vi "DXYN.vi"(11 "Variables and Memory in":T1 {"GFX" format="%02x"}) -> (3 "Variables and Memory out":T1 {"GFX" format="%02x"})   [LabVIEW 2018]
uses:
  Controls/ClusterF.ctl
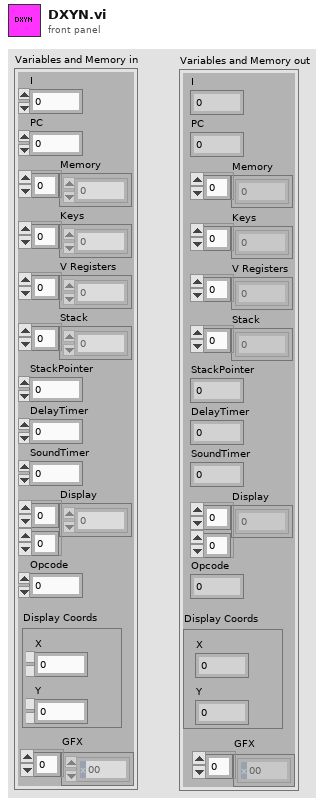
[diagram p1: front panel]
types:
  T1 = typedef "ClusterF.ctl" = cluster{"I":u16, "PC":u16, "Memory":u8[], "Keys":u8[], "V Registers":u8[], "Stack":u16[], "StackPointer":u16, "DelayTimer":u8, "SoundTimer":u8, "Display":u8[][], "Opcode":u16, "Display Coords":cluster{"X":u8, "Y":u8}, "GFX":u8[]}
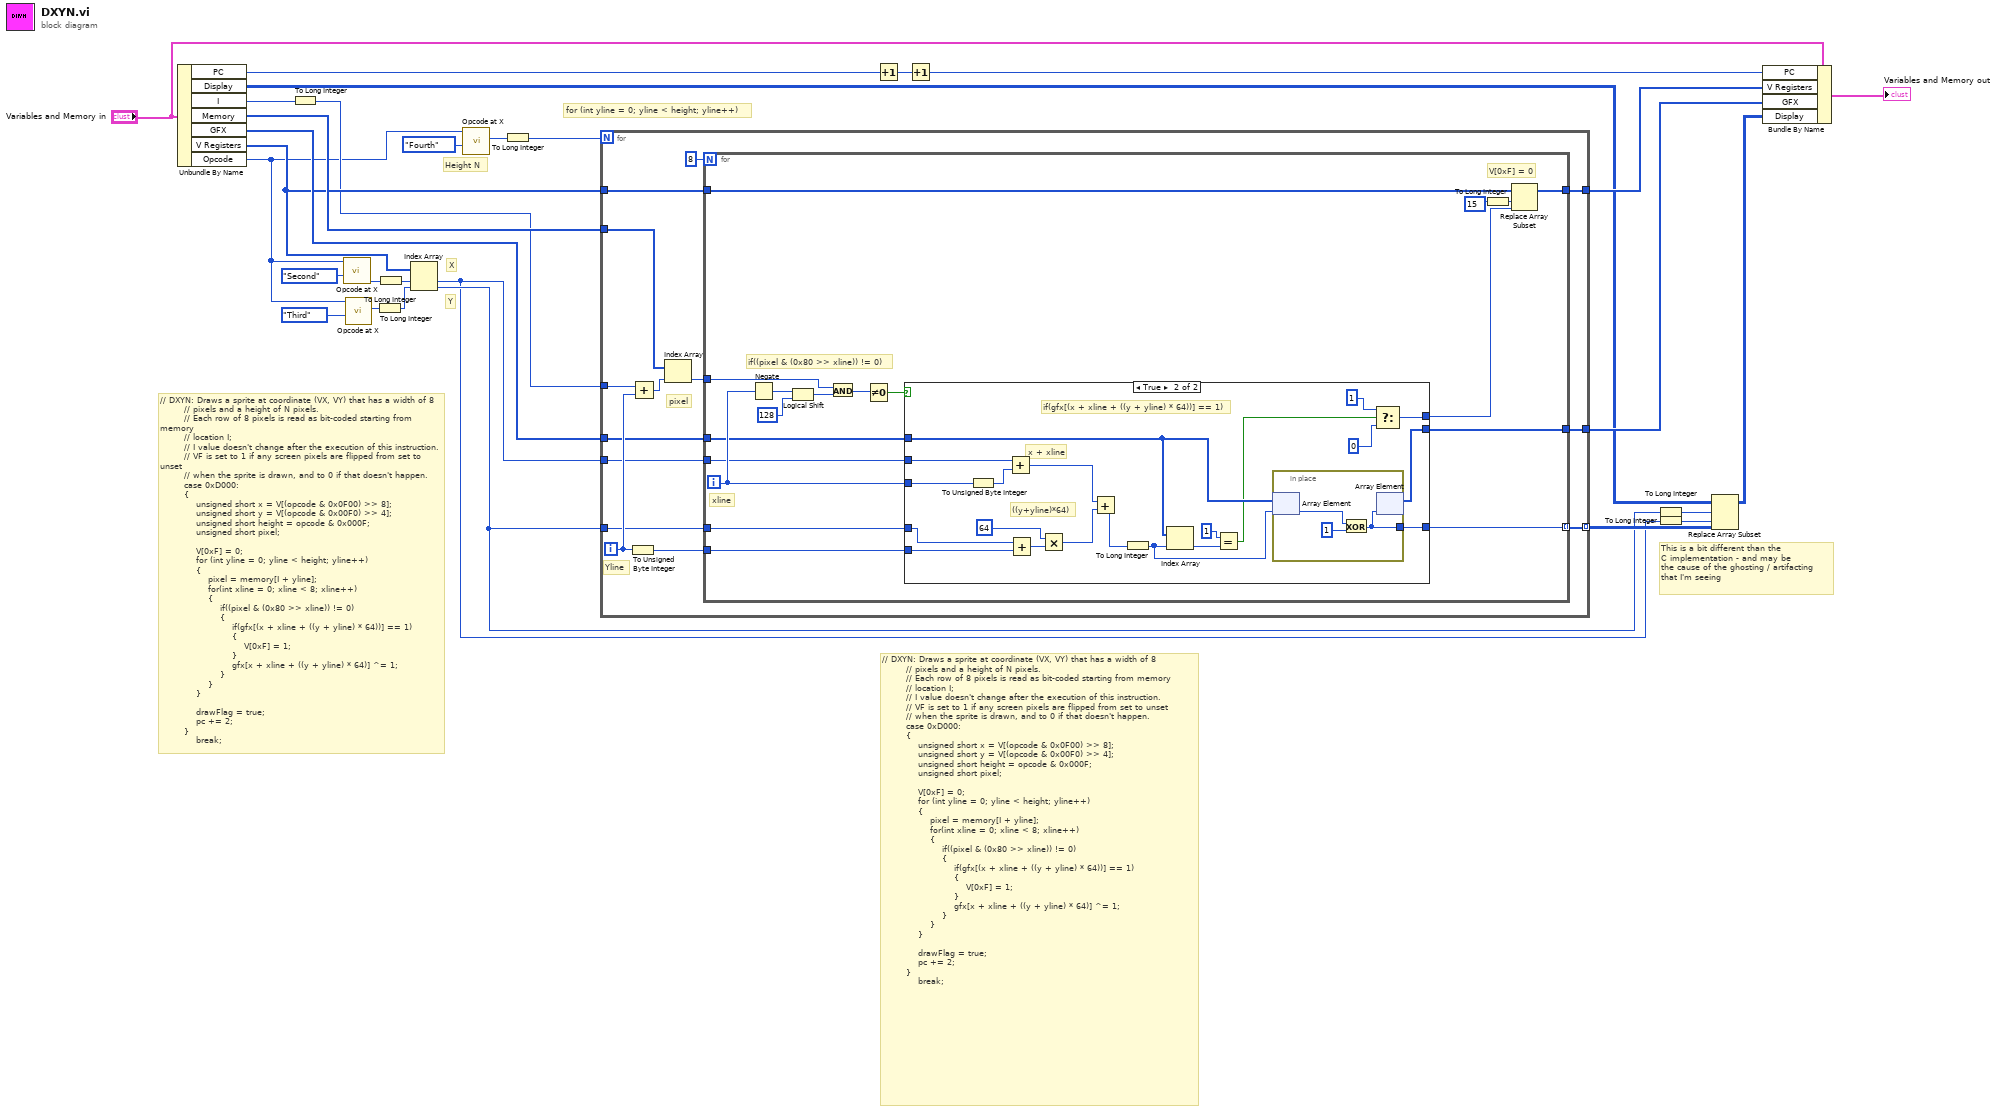
[diagram p0: block diagram]
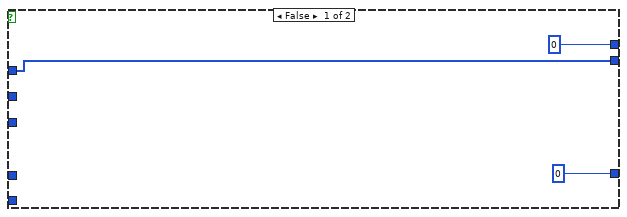
[diagram p2: hidden frame]
diagram:
  # "This is a bit different than the\nC implementation - and may be \nthe cause of the ghosting / artifacting\nthat I'm seeing"
  # "// DXYN: Draws a sprite at coordinate (VX, VY) that has a width of 8\n        // pixels and a height of N pixels.\n        // Each row of 8 pixels is read as bit-coded starting from memory\n        // location I;\n        // I value doesn't change after the execution of this instruction.\n        // VF is set to 1 if any screen pixels are flipped from set to unset\n        // when the sprite is drawn, and to 0 if that doesn't happen.\n        case 0xD000:\n        {\n            unsigned short x = V[(opcode & 0x0F00) >> 8];\n            unsigned short y = V[(opcode & 0x00F0) >> 4];\n            unsigned short height = opcode & 0x000F;\n            unsigned short pixel;\n\n            V[0xF] = 0;\n            for (int yline = 0; yline < height; yline++)\n            {\n                pixel = memory[I + yline];\n                for(int xline = 0; xline < 8; xline++)\n                {\n                    if((pixel & (0x80 >> xline)) != 0)\n                    {\n                        if(gfx[(x + xline + ((y + yline) * 64))] == 1)\n                        {\n                            V[0xF] = 1;\n                        }\n                        gfx[x + xline + ((y + yline) * 64)] ^= 1;\n                    }\n                }\n            }\n\n            drawFlag = true;\n            pc += 2;\n        }\n            break;"
  # "X"
  # "Y"
  # "for (int yline = 0; yline < height; yline++)"
  # "Height N"
  # "// DXYN: Draws a sprite at coordinate (VX, VY) that has a width of 8\n        // pixels and a height of N pixels.\n        // Each row of 8 pixels is read as bit-coded starting from memory\n        // location I;\n        // I value doesn't change after the execution of this instruction.\n        // VF is set to 1 if any screen pixels are flipped from set to unset\n        // when the sprite is drawn, and to 0 if that doesn't happen.\n        case 0xD000:\n        {\n            unsigned short x = V[(opcode & 0x0F00) >> 8];\n            unsigned short y = V[(opcode & 0x00F0) >> 4];\n            unsigned short height = opcode & 0x000F;\n            unsigned short pixel;\n\n            V[0xF] = 0;\n            for (int yline = 0; yline < height; yline++)\n            {\n                pixel = memory[I + yline];\n                for(int xline = 0; xline < 8; xline++)\n                {\n                    if((pixel & (0x80 >> xline)) != 0)\n                    {\n                        if(gfx[(x + xline + ((y + yline) * 64))] == 1)\n                        {\n                            V[0xF] = 1;\n                        }\n                        gfx[x + xline + ((y + yline) * 64)] ^= 1;\n                    }\n                }\n            }\n\n            drawFlag = true;\n            pc += 2;\n        }\n            break;"
  n1 = Unbundle By Name("Variables and Memory in") -> ("PC"=w21:u16, "Display"=w2:u8[][], "I"=w12:u16, "Memory"=w25:u8[], "GFX"=w26:u8[], "V Registers"=w23:u8[], "Opcode"=w8:u16)
  n2 = To Long Integer(number=w12) -> (32bit integer=w9:i32)
  n3 = call "Opcode at X.vi"("X Position"=enum16{"First", "Second", "Third", "Fourth"}."Second", "Opcode"=w8) -> ("Opcode at X Position (U8)"=w15:u8)  [unwired: 9 in]
  n4 = call "Opcode at X.vi"("X Position"=enum16{"First", "Second", "Third", "Fourth"}."Third", "Opcode"=w8) -> ("Opcode at X Position (U8)"=w13:u8)  [unwired: 9 in]
  n5 = To Long Integer(number=w13) -> (32bit integer=w7:i32)
  n6 = To Long Integer(number=w15) -> (32bit integer=w14:i32)
  n7 = Index Array(array=w23, index #1=w14, index #2=w7) -> (element #1=w5:u8, element #2=w6:u8)
  n8 = call "Opcode at X.vi"("X Position"=enum16{"First", "Second", "Third", "Fourth"}."Fourth", "Opcode"=w8) -> ("Opcode at X Position (U8)"=w11:u8)  [unwired: 9 in]
  n9 = To Long Integer(number=w11) -> (32bit integer=w24:i32)
  n10 = for {
    N: w24 -> [_]
    tunnel: w23 -> [w43]
    tunnel: w26 -> [w38]
    tunnel: w6 -> [w36]
    tunnel: w5 -> [w35]
    tunnel: w25 -> [w41]
    tunnel: [w34] -> w28
    tunnel: w9 -> [w33]
    tunnel: [w32] -> w27
    tunnel: [w30] -> w29 mode=indexing
    i -> [w40]
    # "pixel"
    # "Yline"
    n11 = To Unsigned Byte Integer(number=w40) -> (unsigned 8bit integer=w37:u8)
    n12 = Add(x=w33, y=w40) -> (x+y=w39:i32)
    n13 = Index Array(array=w41, index=w39) -> (element=w31:u8)
    n14 = for {
      N: 8 -> [_]
      tunnel: w43 -> [w59]
      tunnel: w31 -> [w57]
      tunnel: w38 -> [w51]
      tunnel: w37 -> [w50]
      tunnel: w36 -> [w49]
      tunnel: w35 -> [w48]
      tunnel: [w46] -> w34
      tunnel: [w45] -> w32
      tunnel: [w44] -> w30 mode=indexing
      i -> [w52]
      # "if((pixel & (0x80 >> xline)) != 0)"
      # "V[0xF] = 0"
      # "xline"
      n15 = Negate(x=w52) -> (-x=w54:i32)
      n16 = Logical Shift(y=w54, x=u8 128 ("y")) -> (x << y=w58:u8)
      n17 = And(x=w57, y=w58) -> (x .and. y?=w56:u8)
      n18 = Not Equal To 0?(x=w56) -> (x != 0?=w53:bool)
      n19 = case shown="True" w53 {
        tunnel: w52 -> [_ w80]
        tunnel: w51 -> [w63 w76]
        tunnel: w50 -> [_ w78]
        tunnel: w49 -> [_ w66]
        tunnel: w48 -> [_ w65]
        tunnel: [u8 0 ("t") w72] -> w47
        tunnel: [w63 w74] -> w46
        tunnel: [u8 0 w67] -> w44
        frame False {
        }
        frame True {
          # "((y+yline)*64)"
          # "x + xline"
          # "if(gfx[(x + xline + ((y + yline) * 64))] == 1)"
          n20 = To Unsigned Byte Integer(number=w80) -> (unsigned 8bit integer=w68:u8)
          n21 = Add(x=w65, y=w68) -> (x+y=w82:u8)
          n22 = Add(x=w66, y=w78) -> (x+y=w81:u8)
          n23 = Multiply(x=u8 64, y=w81) -> (x*y=w83:u8)
          n24 = Add(x=w82, y=w83) -> (x+y=w84:u8)
          n25 = To Long Integer(number=w84) -> (32bit integer=w75:i32)
          n26 = Index Array(array=w76, index=w75) -> (element=w77:u8)
          n27 = Equal?(x=u8 1, y=w77) -> (x = y?=w73:bool)
          n28 = in-place {
            in-place-border: [w85] -> w67
            n29 = in-place-array #1(w76, w75) -> (w87:u8)
            n30 = Exclusive Or(1:u8 1 ("y"), 2:w87) -> (0:w85:u8)
            n31 = in-place-array #1(w85) -> (w74:u8[])  [unwired: 1 out]
          }
          n32 = Select(t=u8 1 ("x"), s=w73, f=u8 0 ("x")) -> (s? t:f=w72:u8)
        }
      }
      n33 = To Long Integer(number=15) -> (32bit integer=w61:i32)
      n34 = Replace Array Subset(array=w59, new element=w47, index=w61) -> (w45:u8[])
    }
  }
  n35 = Increment(x=w21) -> (x+1=w20:u16)
  n36 = Increment(x=w20) -> (x+1=w22:u16)
  n37 = To Long Integer(number=w6) -> (32bit integer=w4:i32)
  n38 = To Long Integer(number=w5) -> (32bit integer=w3:i32)
  n39 = Replace Array Subset(array=w2, new element=w29, index (row)=w4, index (col)=w3) -> (w1:u8[][])
  n40 = Bundle By Name(cluster="Variables and Memory in", "PC"=w22, "V Registers"=w27, "GFX"=w28, "Display"=w1) -> (→"Variables and Memory out":T1)
